vi "configureNumberOfValues.vi"(11 "TDMS File Viewer Configuration":T1) -> (3 "TDMS File Viewer Configuration Out":T1)   [LabVIEW 2017]
uses:
  <vilib>/Utility/tdmsutil.llb/fileViewerConfigData.ctl
panel:
  in  "Help":bool
  in  "Starting at":u64=1000
  in  "Starting at":u64=1000
  in  "Cancel":bool
  in  "Ok":bool
  in  "no show":bool
  in  "Number of values":u64=100000
  in  "Number of values (graph)":enum32{"ALL", "Limited"}(radio)
  in  "Number of values":u64=1000
  in  "Number of values (table)":enum32{"ALL", "Limited"}(radio)
  # "Number of values to load"
  # "You are trying to load a large amount of data. Loading and displaying that data can take up to several minutes. Very large waveforms might also not fit into the memory of your computer."
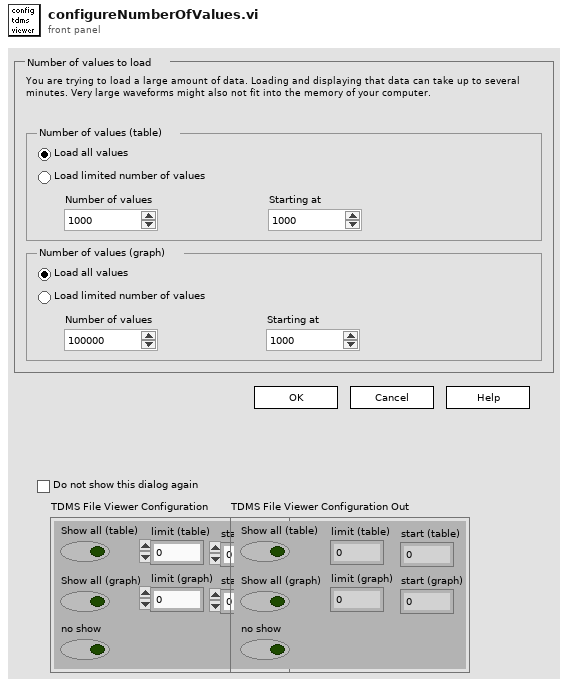
[diagram p1: front panel]
types:
  T1 = typedef "fileViewerConfigData.ctl" = cluster{"Show all (table)":bool, "Show all (graph)":bool, "limit (table)":u64, "limit (graph)":u64, "no show":bool, "start (table)":u64, "start (graph)":u64}
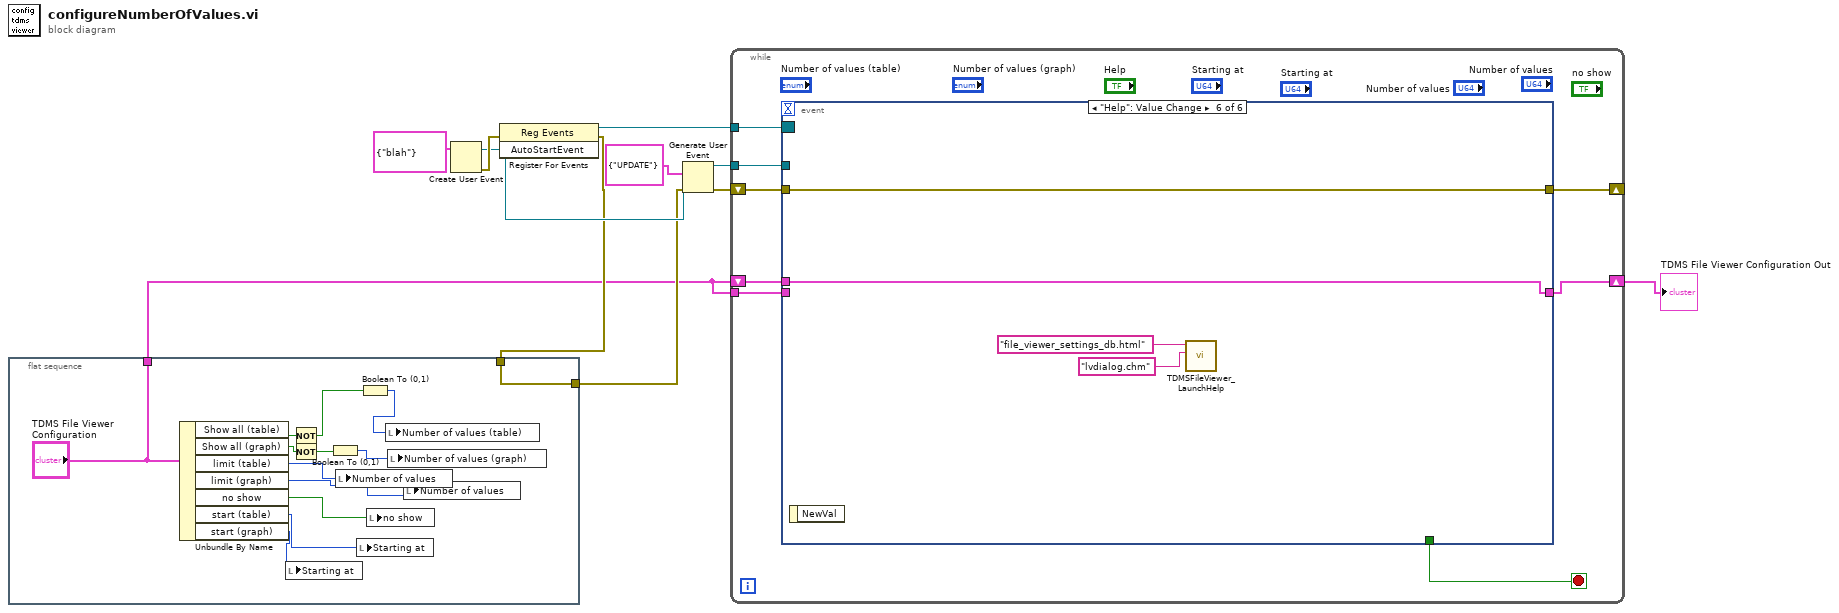
[diagram p0: block diagram]
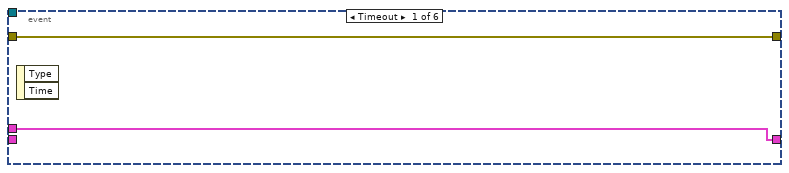
[diagram p2: hidden frame]
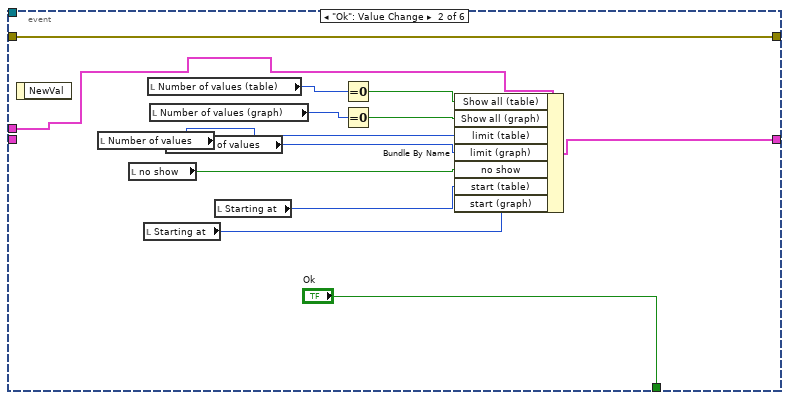
[diagram p3: hidden frame]
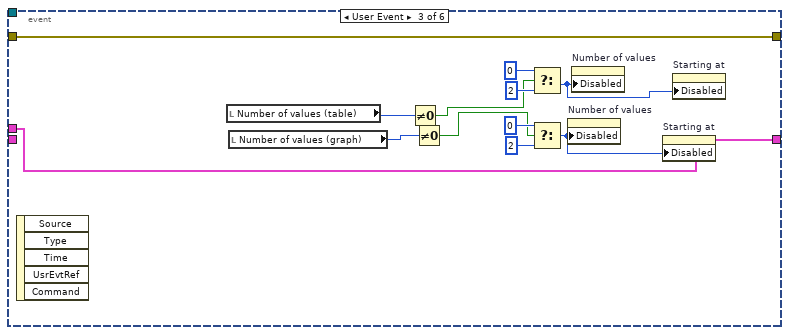
[diagram p4: hidden frame]
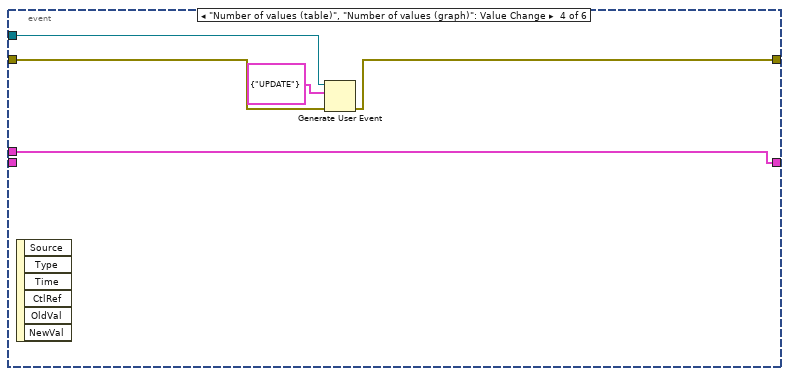
[diagram p5: hidden frame]
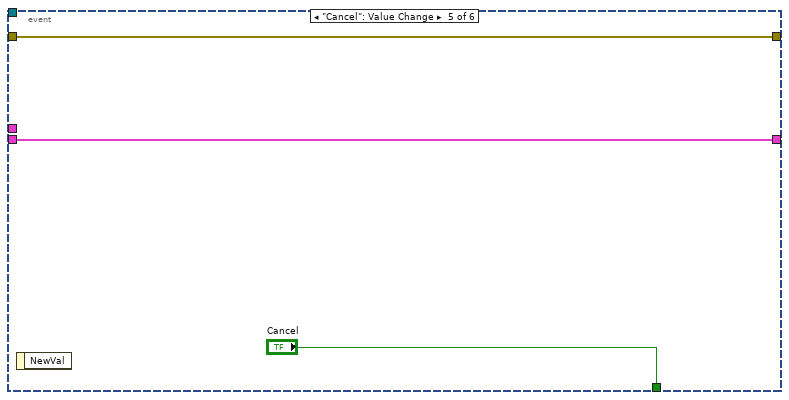
[diagram p6: hidden frame]
diagram:
  n1 = flat-sequence {
    tunnel: w4 -> [w19]
    tunnel: [w19] -> w3
    tunnel: ["TDMS File Viewer Configuration"] -> w1
    frame #0 {
      n2 = Unbundle By Name("TDMS File Viewer Configuration") -> ("Show all (table)"=w15:bool, "Show all (graph)"=w12:bool, "limit (table)"=w23:u64, "limit (graph)"=w24:u64, "no show"=w21:bool, "start (table)"=w17:u64, "start (graph)"=w16:u64)
      n3 = local write "Starting at"(w16) -> ()
      n4 = Not(x=w15) -> (.not. x?=w14:bool)
      n5 = Not(x=w12) -> (.not. x?=w13:bool)
      n6 = Boolean To (0,1)(Boolean=w13) -> (0, 1=w22:i16)
      n7 = local write "Number of values"(w23) -> ()
      n8 = local write "Starting at"(w17) -> ()
      n9 = Boolean To (0,1)(Boolean=w14) -> (0, 1=w20:i16)
      n10 = local write "no show"(w21) -> ()
      n11 = local write "Number of values (table)"(w20) -> ()
      n12 = local write "Number of values (graph)"(w22) -> ()
      n13 = local write "Number of values"(w24) -> ()
    }
  }
  n14 = Create User Event(user event datatype=cluster{"Command":string} {"Command"="blah"} ("AutoStartEvent")) -> (user event=w6:refnum<user-event>, error out=w8:errorcluster)  [unwired: 1 in]
  n15 = register-events(error in=w8, w6) -> (reference out=w9:refnum<event-registration>, error out=w4:errorcluster)  [unwired: 1 in]
  n16 = Generate User Event(user event=w6, event data cluster=cluster{"Action":string} {"Action"="UPDATE"} ("event data"), error in=w3) -> (user event out=w5:refnum<user-event>, error out=w7:errorcluster)  [unwired: 1 in]
  n17 = while {
    tunnel: w9 -> [w31]
    shift-right: [w29] -> _
    shift-left: w7 -> [w30]
    tunnel: w5 -> [w28]
    shift-right: [w27] -> w2
    shift-left: w1 -> [w26]
    tunnel: w1 -> [w25]
    stop <- w32 stop-if-true
    n18 = event shown="[5] \"Help\": Value Change" {
      selector: w31 -> [_ _ _ _ _ _]
      dyn-events: _ -> [_ _ _ _ _ _]
      timeout: _ -> [_ _ _ _ _ _]
      tunnel: [_ "Ok" _ _ "Cancel" _] -> w32
      tunnel: w30 -> [w34 w46 w59 w63 w66 w70]
      tunnel: [w34 w46 w59 w62 w66 w70] -> w29
      tunnel: w28 -> [_ _ _ w61 _ _]
      tunnel: [w33 w38 w50 w60 w65 w71] -> w27
      tunnel: w26 -> [w33 w37 w50 w60 _ w71]
      tunnel: w25 -> [_ _ _ _ w65 _]
      event Timeout {
        n19 = event-data() -> ()  [unwired: 1 in, 2 out]
      }
      event "Ok": Value Change {
        n20 = event-data() -> ()  [unwired: 1 in, 1 out]
        n21 = local read "Number of values"() -> (w40:u64)
        n22 = local read "no show"() -> (w39:bool)
        n23 = local read "Starting at"() -> (w35:u64)
        n24 = local read "Number of values (table)"() -> (w45:enum32{"ALL", "Limited"})
        n25 = local read "Number of values (graph)"() -> (w43:enum32{"ALL", "Limited"})
        n26 = local read "Number of values"() -> (w41:u64)
        n27 = local read "Starting at"() -> (w36:u64)
        n28 = Equal To 0?(x=w45) -> (x = 0?=w44:bool)
        n29 = Equal To 0?(x=w43) -> (x = 0?=w42:bool)
        n30 = Bundle By Name(cluster=w37, "Show all (table)"=w44, "Show all (graph)"=w42, "limit (table)"=w40, "limit (graph)"=w41, "no show"=w39, "start (table)"=w36, "start (graph)"=w35) -> (w38:T1)
      }
      event User Event {
        n31 = event-data() -> ()  [unwired: 1 in, 5 out]
        n32 = local read "Number of values (table)"() -> (w54:enum32{"ALL", "Limited"})
        n33 = local read "Number of values (graph)"() -> (w53:enum32{"ALL", "Limited"})
        n34 = Not Equal To 0?(x=w54) -> (x != 0?=w51:bool)
        n35 = Not Equal To 0?(x=w53) -> (x != 0?=w52:bool)
        n36 = Select(t=0, s=w51, f=2 ("t")) -> (s? t:f=w49:i32)
        n37 = Select(t=0, s=w52, f=2 ("t")) -> (s? t:f=w48:i32)
        n38 = property on="Number of values" class="DigNum (strict)"("Disabled"=w48) -> ()  [unwired: 2 in, 2 out]
        n39 = property on="Number of values" class="DigNum (strict)"("Disabled"=w49) -> ()  [unwired: 2 in, 2 out]
        n40 = property on="Starting at" class="DigNum (strict)"("Disabled"=w48) -> ()  [unwired: 2 in, 2 out]
        n41 = property on="Starting at" class="DigNum (strict)"("Disabled"=w49) -> ()  [unwired: 2 in, 2 out]
      }
      event "Number of values (table)", "Number of values (graph)": Value Change {
        n42 = event-data() -> ()  [unwired: 1 in, 6 out]
        n43 = Generate User Event(user event=w61, event data cluster=cluster{"Action":string} {"Action"="UPDATE"} ("event data"), error in=w63) -> (error out=w62:errorcluster)  [unwired: 1 in, 1 out]
      }
      event "Cancel": Value Change {
        n44 = event-data() -> ()  [unwired: 1 in, 1 out]
      }
      event "Help": Value Change {
        n45 = event-data() -> ()  [unwired: 1 in, 1 out]
        n46 = call <vilib>:"TDMSFileViewer_LaunchHelp.vi"("CHM or HLP filename (lvdialog.chm)"="lvdialog.chm", "HTML filename"="file_viewer_settings_db.html") -> ()  [unwired: 1 in, 5 out]
      }
    }
  }
  "TDMS File Viewer Configuration Out" <- w2
